vi "Check_Presence_of_Connected_Tracks-2.vi"(3 "error IN":errorcluster, 4 "[IN] #of Frames":i32, 5 "[IN] Still connected\ntracks in group":T1) -> (0 "error OUT":errorcluster, 2 "[OUT] At least two tracks\ninside track group":bool)   [LabVIEW 2013]
doc: "This subprogram checks the existence of at least two connected points in a group of tracks (for making further iterations for conflicts resolving)"
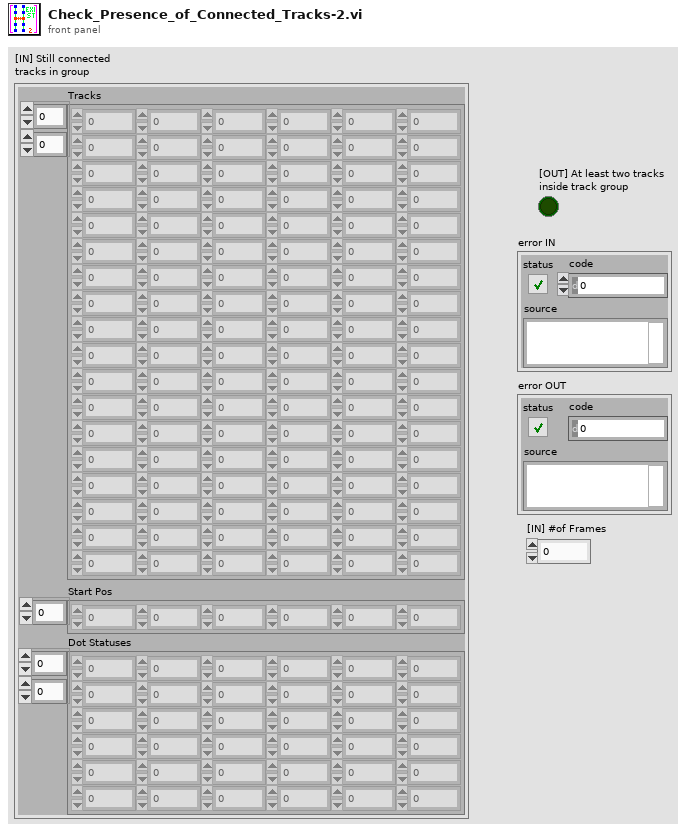
[diagram p1: front panel]
types:
  T1 = cluster{"Tracks":dbl[][], "Start Pos":i32[], "Dot Statuses":i16[][]}
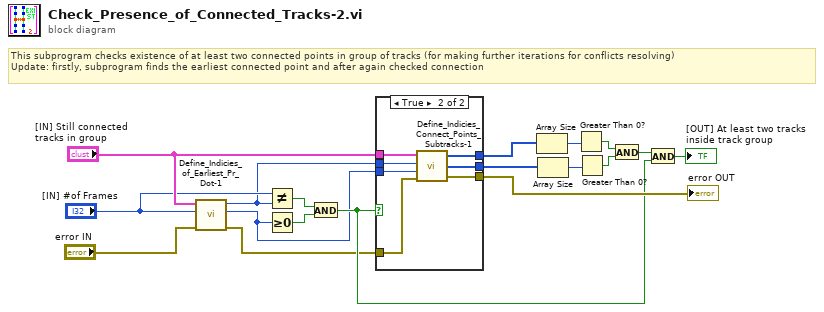
[diagram p0: block diagram]
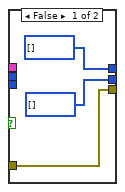
[diagram p2: hidden frame]
diagram:
  # "This subprogram checks existence of at least two connected points in group of tracks (for making further iterations for conflicts resolving)\nUpdate: firstly, subprogram finds the earliest connected point and after again checked connection"
  n1 = call "Define_Indicies_of_Earliest_Pr_Dot-1.vi"("error IN"="error IN", "[IN] #of Frames"="[IN] #of Frames", "[IN] Still connected\ntracks in group"="[IN] Still connected\ntracks in group") -> ("error OUT"=w3:errorcluster, "[OUT] Index of Subtrack"=w1:i32, "[OUT] Index of Ear\nliest Problem Point"=w2:i32)  [unwired: 2 in]
  n2 = Not Equal?(x="[IN] #of Frames", y=w2) -> (x != y?=w4:bool)
  n3 = Greater Or Equal To 0?(x=w1) -> (x >= 0?=w18:bool)
  n4 = And(x=w4, y=w18) -> (x .and. y?=w12:bool)
  n5 = case shown="True" w12 {
    tunnel: "[IN] Still connected\ntracks in group" -> [_ w28]
    tunnel: [w19 w25] -> w14
    tunnel: [i32[] [] ("[OUT] Index of \nconnected dots\ninside the track") w26] -> w17
    tunnel: [i32[] [] ("[OUT] Index of connected\ntracks with problem dot") w27] -> w9
    tunnel: w3 -> [w19 w24]
    tunnel: w2 -> [_ w23]
    tunnel: w1 -> [_ w22]
    frame False {
    }
    frame True {
      n6 = call "Define_Indicies_Connect_Points_Subtracks-1.vi"("error IN"=w24, "[IN] Index of track with\n(problem displacement)"=w22, "[IN] Index of problem\ndisplacement inside track"=w23, "[IN] Track group"=w28) -> ("error OUT"=w25:errorcluster, "[OUT] Index of \nconnected dots\ninside the track"=w26:i32[], "[OUT] Index of connected\ntracks with problem dot"=w27:i32[])
    }
  }
  "error OUT" <- w14
  n7 = Array Size(array=w9) -> (size(s)=w10:i32)
  n8 = Array Size(array=w17) -> (size(s)=w16:i32)
  n9 = Greater Than 0?(x=w10) -> (x > 0?=w8:bool)
  n10 = Greater Than 0?(x=w16) -> (x > 0?=w15:bool)
  n11 = And(x=w8, y=w15) -> (x .and. y?=w13:bool)
  n12 = And(x=w13, y=w12) -> (x .and. y?=→"[OUT] At least two tracks\ninside track group":bool)
